vi "Write All Child Attributes.vi"(10 "All Child Attributes":T1, 11 "Base Actor in":refnum<class "Base Actor.lvclass">) -> (3 "Base Actor out":refnum<class "Base Actor.lvclass">)   [LabVIEW 2025, in "jettl.lvlib" / "Base Actor.lvlib" / "Base Actor.lvclass"]
uses:
  Base Actor.lvclass
  All Child Attributes.ctl
  Attributes/Attributes.lvclass
  Base Actor.lvclass/Base Actor.ctl
  jettl.lvlib
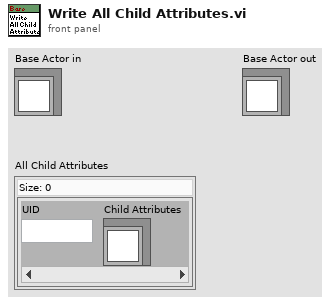
[diagram p1: front panel]
types:
  T1 = typedef "jettl.lvlib/All Child Attributes.ctl" = map{string, refnum<class "Attributes.lvclass">}
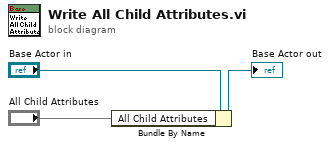
[diagram p0: block diagram]
diagram:
  n1 = Bundle By Name(cluster="Base Actor in", "All Child Attributes"="All Child Attributes") -> (→"Base Actor out":refnum<class "Base Actor.lvclass">)
